vi "test_F9P-fgv.vi"() -> ()   [LabVIEW 2019]
uses:
  Ctrl/gnss_config.ctl
panel:
  out "error out":errorcluster
  out "read_buffer":string
  in  "GNSS cfg":T1={"Port"="COM10", "heading select"="", "PwrPak7_mode select"=[], "rate"=115200}
  out "UTM graph":cluster{"X":dbl, "Y":dbl}[](graph)=[{"X"=161777.95400057395, "Y"=515289.5740891766}, {"X"=161777.91880889426, "Y"=515289.640840397}, {"X"=161777.91926328043, "Y"=515289.74072502257}, {"X"=161777.89309671233, "Y"=515289.8407307517}, {"X"=161777.83123359273, "Y"=515289.89650478243}, {"X"=161777.8049155659, "Y"=515289.96321563463}, {"X"=161777.78731972742, "Y"=515289.99659124424}, {"X"=161777.7073558953, "Y"=515289.97475796775}, {"X"=161777.6717603178, "Y"=515289.95272285305}, {"X"=161777.59169550939, "Y"=515289.90869299456}, {"X"=161777.53835263004, "Y"=515289.8867386161}, {"X"=161777.5565543218, "Y"=515289.98654250597}, {"X"=161777.94820664724, "Y"=515290.2511253461}, {"X"=161778.5442558229, "Y"=515290.58136952063}, {"X"=161779.19379927934, "Y"=515290.9668630023}, {"X"=161779.82615070668, "Y"=515291.4745184741}, {"X"=161780.5468851608, "Y"=515291.90408230544}, {"X"=161781.3293312115, "Y"=515292.24457731773}, {"X"=161782.0763330891, "Y"=515292.5963321432}, {"X"=161782.7433711131, "Y"=515292.92625371326}, {"X"=161783.43763578677, "Y"=515293.3892337531}, {"X"=161784.1312441562, "Y"=515293.707936055}, {"X"=161784.81607978063, "Y"=515294.04887535865}, {"X"=161785.45700141956, "Y"=515294.4899011407}, {"X"=161786.09792298873, "Y"=515294.93092697154}, {"X"=161786.7387940146, "Y"=515295.3608545599}, {"X"=161787.44137668586, "Y"=515295.70171335887}, {"X"=161788.13513613178, "Y"=515296.0537108666}, {"X"=161788.81114823182, "Y"=515296.4057891417}, {"X"=161789.51388214662, "Y"=515296.7799429905}, {"X"=161790.16377791404, "Y"=515297.24312535825}, {"X"=161790.75927092956, "Y"=515297.4512891845}, {"X"=161791.45222257613, "Y"=515297.6257142923}, {"X"=161792.2164661421, "Y"=515297.8664063941}, {"X"=161792.9802554574, "Y"=515298.00721393456}, {"X"=161793.57564741094, "Y"=515298.1931813774}, {"X"=161794.04680835863, "Y"=515298.3797137626}, {"X"=161794.66105778705, "Y"=515298.8097630031}, {"X"=161795.2851396199, "Y"=515299.4506394842}, {"X"=161795.79295568907, "Y"=515299.8922712862}, {"X"=161796.44179114, "Y"=515300.1223900075}, {"X"=161797.13539845136, "Y"=515300.4410933779}, {"X"=161797.67023897104, "Y"=515300.97139058786}, {"X"=161798.35436699775, "Y"=515301.1569549014}, {"X"=161799.0217064507, "Y"=515301.5534675081}, {"X"=161799.63580401638, "Y"=515301.95022223337}, {"X"=161800.4886824086, "Y"=515302.168315055}, {"X"=161801.34135892912, "Y"=515302.3420147952}, {"X"=161802.02755544466, "Y"=515302.98260937684}, {"X"=161802.80137821336, "Y"=515303.37863818085}, {"X"=161803.5310850009, "Y"=515303.83036021655}, {"X"=161804.18138306442, "Y"=515304.3823299997}, {"X"=161804.83979789636, "Y"=515304.7677851127}, {"X"=161805.60444402587, "Y"=515305.0972647629}, {"X"=161806.39525694898, "Y"=515305.3267388399}, {"X"=161807.21314476756, "Y"=515305.6559766089}, {"X"=161807.87039905335, "Y"=515305.7861712441}, {"X"=161808.54550148163, "Y"=515305.9384818447}, {"X"=161809.22151191556, "Y"=515306.29056175554}, {"X"=161809.90669859963, "Y"=515306.70919113874}, {"X"=161810.5830115807, "Y"=515307.12786090834}, {"X"=161811.30308733214, "Y"=515307.41314957023}, {"X"=161812.0322888786, "Y"=515307.7538894202}, {"X"=161812.72589495758, "Y"=515308.0725940717}, {"X"=161813.28574078486, "Y"=515308.2476259363}, {"X"=161813.93437333827, "Y"=515308.43335283204}, {"X"=161814.49391648162, "Y"=515308.54179502284}, {"X"=161814.78750287872, "Y"=515308.7069385592}, {"X"=161814.86736555945, "Y"=515308.70657560363}, {"X"=161814.89428908148, "Y"=515308.7730443711}, {"X"=161814.89474303092, "Y"=515308.87292899843}, {"X"=161814.9569593225, "Y"=515308.89484328456}, {"X"=161814.98358021321, "Y"=515308.8947222998}, {"X"=161815.0456956249, "Y"=515308.89444000245}, {"X"=161815.0901646555, "Y"=515308.9164349459}, {"X"=161815.14370907008, "Y"=515308.9827827293}, {"X"=161815.2241770044, "Y"=515309.1155992807}, {"X"=161815.30444318076, "Y"=515309.2040226664}, {"X"=161815.39373430205, "Y"=515309.3257005998}, {"X"=161815.4736978485, "Y"=515309.34753423324}, {"X"=161815.52704050532, "Y"=515309.36948885216}, {"X"=161815.58033272164, "Y"=515309.38034517795}, {"X"=161815.64270031895, "Y"=515309.4355543454}, {"X"=161815.68711890728, "Y"=515309.44645099895}, {"X"=161815.7316888065, "Y"=515309.4906425299}, {"X"=161815.7674355156, "Y"=515309.54597268056}, {"X"=161815.8119549762, "Y"=515309.57906591985}, {"X"=161815.85632312373, "Y"=515309.57886428316}, {"X"=161815.89186808158, "Y"=515309.58980126516}, {"X"=161815.92741303705, "Y"=515309.6007382487}, {"X"=161815.95398349033, "Y"=515309.5895189744}, {"X"=161815.90916140308, "Y"=515309.48983598285}, {"X"=161815.93598404175, "Y"=515309.5341081699}, {"X"=161815.95378174057, "Y"=515309.54512580705}, {"X"=161815.97147856222, "Y"=515309.53394686105}, {"X"=161815.98040262918, "Y"=515309.54500482546}, {"X"=161816.0160988968, "Y"=515309.58923668414}, {"X"=161816.06076966808, "Y"=515309.65562480193}, {"X"=161816.18520223314, "Y"=515309.6994533913}, {"X"=161816.22982256542, "Y"=515309.754743216}, {"X"=161816.26521620865, "Y"=515309.73238532426}, {"X"=161816.30055941732, "Y"=515309.6989291415}, {"X"=161816.32738205325, "Y"=515309.74320132786}, {"X"=161816.18449611322, "Y"=515309.5440773027}, {"X"=161816.11305313953, "Y"=515309.4445152901}, {"X"=161816.13080039885, "Y"=515309.44443463604}, {"X"=161816.14885028123, "Y"=515309.51094373537}, {"X"=161816.1668497262, "Y"=515309.5663545408}, {"X"=161816.25639301635, "Y"=515309.7435239428}, {"X"=161816.51468657114, "Y"=515309.95322201477}, {"X"=161817.0042996991, "Y"=515310.29505111795}, {"X"=161817.65373897512, "Y"=515310.65835097386}, {"X"=161818.44465190032, "Y"=515310.9100227651}, {"X"=161819.26248826162, "Y"=515311.2281634111}, {"X"=161820.07099704226, "Y"=515311.44645983004}, {"X"=161820.90537020008, "Y"=515311.49816098064}, {"X"=161821.74896998494, "Y"=515311.6275099376}, {"X"=161822.53917668908, "Y"=515311.723806025}, {"X"=161823.3205601771, "Y"=515311.83124079654}, {"X"=161824.10229662905, "Y"=515312.01636368537}, {"X"=161824.87546197322, "Y"=515312.2681167172}, {"X"=161825.6757019711, "Y"=515312.6196334966}, {"X"=161826.44004401113, "Y"=515312.8825252806}, {"X"=161827.20433557767, "Y"=515313.13431884075}, {"X"=161828.02186885226, "Y"=515313.38587058336}, {"X"=161828.82180608835, "Y"=515313.6707979099}, {"X"=161829.66601055447, "Y"=515313.9333271637}, {"X"=161830.48324116512, "Y"=515314.11828939256}, {"X"=161831.35401598827, "Y"=515314.3695995875}, {"X"=161832.19837155048, "Y"=515314.665423971}, {"X"=161833.016559914, "Y"=515315.0612539941}, {"X"=161833.74565907218, "Y"=515315.37979913654}, {"X"=161834.43921326537, "Y"=515315.68740728305}, {"X"=161835.15933786728, "Y"=515315.9837962724}, {"X"=161835.89726006903, "Y"=515316.2912030018}, {"X"=161836.63518221842, "Y"=515316.598609796}, {"X"=161837.37320513173, "Y"=515316.9282132381}, {"X"=161838.10245518197, "Y"=515317.2800536338}, {"X"=161838.8584268477, "Y"=515317.65396976646}, {"X"=161839.62352409755, "Y"=515318.083337126}, {"X"=161840.30830503887, "Y"=515318.4131826406}, {"X"=161841.0286812179, "Y"=515318.76506358985}, {"X"=161841.77557738448, "Y"=515319.09462711634}, {"X"=161842.54042233957, "Y"=515319.46850327816}, {"X"=161843.24350470793, "Y"=515319.9203496465}, {"X"=161843.9554606182, "Y"=515320.3721557716}, {"X"=161844.631921982, "Y"=515320.82412314625}, {"X"=161845.31725688517, "Y"=515321.2760502795}, {"X"=161846.07312706957, "Y"=515321.6277704748}, {"X"=161846.81967000206, "Y"=515321.8796464045}, {"X"=161847.59273294985, "Y"=515322.1092049326}, {"X"=161848.31280612783, "Y"=515322.3944967517}, {"X"=161849.10391857562, "Y"=515322.6905645844}, {"X"=161849.85025974846, "Y"=515322.8980476132}, {"X"=161850.52480569232, "Y"=515322.92828036164}, {"X"=161851.28864208458, "Y"=515323.0801914752}, {"X"=161852.08802329528, "Y"=515323.24303979415}, {"X"=161852.87011074505, "Y"=515323.5058533946}, {"X"=161853.64337491884, "Y"=515323.7798056455}, {"X"=161854.3632461972, "Y"=515324.02070481237}, {"X"=161855.10988943258, "Y"=515324.2947780592}, {"X"=161855.89222861396, "Y"=515324.61308340123}, {"X"=161856.67471888705, "Y"=515324.9646836894}, {"X"=161857.47475478542, "Y"=515325.27181031683}, {"X"=161858.2394473211, "Y"=515325.61239302583}, {"X"=161858.96017477982, "Y"=515326.0419635504}, {"X"=161859.69834711196, "Y"=515326.40486382256}, {"X"=161860.5074578888, "Y"=515326.7563436241}, {"X"=161861.28954474037, "Y"=515327.0191580045}, {"X"=161862.02746499534, "Y"=515327.32656702003}, {"X"=161862.76538520248, "Y"=515327.63397609856}, {"X"=161863.53002692718, "Y"=515327.9634609943}, {"X"=161864.29471896973, "Y"=515328.30404425325}, {"X"=161865.06818381284, "Y"=515328.6223907203}, {"X"=161865.84164859212, "Y"=515328.94073725946}, {"X"=161866.57049341834, "Y"=515329.20379377867}, {"X"=161867.33488300277, "Y"=515329.47778755915}, {"X"=161868.09937327213, "Y"=515329.7739779929}, {"X"=161868.82877200074, "Y"=515330.1591159194}, {"X"=161869.56709463586, "Y"=515330.5553119311}, {"X"=161870.3317861905, "Y"=515330.8958957367}, {"X"=161871.06133581288, "Y"=515331.31432873226}, {"X"=161871.80873330153, "Y"=515331.7548778398}, {"X"=161872.52078738002, "Y"=515332.22888295737}, {"X"=161873.2063716484, "Y"=515332.73630381504}, {"X"=161873.8827800619, "Y"=515333.1771752419}, {"X"=161874.57688525325, "Y"=515333.60686789843}, {"X"=161875.27094001378, "Y"=515334.02546231856}, {"X"=161876.06215110896, "Y"=515334.3437292654}, {"X"=161876.7820711783, "Y"=515334.59572863765}, {"X"=161877.53773739794, "Y"=515334.90305848164}, {"X"=161878.1777949538, "Y"=515335.15542033466}, {"X"=161878.83554931934, "Y"=515335.39660342183}, {"X"=161879.61758442305, "Y"=515335.6483212079}, {"X"=161880.42618993216, "Y"=515335.8888199965}, {"X"=161881.31536272637, "Y"=515336.2843326286}, {"X"=161882.11595047737, "Y"=515336.713542806}, {"X"=161882.925109656, "Y"=515337.0761230474}, {"X"=161883.8140808093, "Y"=515337.42724277306}, {"X"=161884.68545573042, "Y"=515337.81173797994}, {"X"=161885.48589212738, "Y"=515338.2076535997}, {"X"=161886.30382391758, "Y"=515338.54799732764}, {"X"=161887.15694797394, "Y"=515338.8215903732}, {"X"=161888.00104734325, "Y"=515339.0619288787}, {"X"=161888.8096522778, "Y"=515339.3024284715}, {"X"=161889.6010133728, "Y"=515339.6539915637}, {"X"=161890.38329944562, "Y"=515339.96120180906}, {"X"=161891.20990310656, "Y"=515340.2571125954}, {"X"=161892.07245413205, "Y"=515340.65274710406}, {"X"=161892.88146147915, "Y"=515340.9820334242}, {"X"=161893.70801461404, "Y"=515341.266846164}, {"X"=161894.51687083603, "Y"=515341.562837765}, {"X"=161895.34337352356, "Y"=515341.8365523713}, {"X"=161896.16115355797, "Y"=515342.1436021796}, {"X"=161896.98760579992, "Y"=515342.40621865366}, {"X"=161897.78743720995, "Y"=515342.668955934}, {"X"=161898.53417799206, "Y"=515342.9652296072}, {"X"=161899.3162621102, "Y"=515343.2280475129}, {"X"=161900.21380354543, "Y"=515343.5125389749}, {"X"=161901.05800270947, "Y"=515343.77507537254}, {"X"=161901.87623526133, "Y"=515344.1820103629}, {"X"=161902.65867142286, "Y"=515344.52251662395}, {"X"=161903.405361544, "Y"=515344.8076924376}, {"X"=161904.1878982269, "Y"=515345.17039542255}, {"X"=161905.05009587965, "Y"=515345.48834321246}, {"X"=161905.8766481465, "Y"=515345.7731571441}, {"X"=161906.73864439924, "Y"=515346.04671193776}, {"X"=161907.60971545277, "Y"=515346.3646197568}, {"X"=161908.4986342502, "Y"=515346.70464379125}, {"X"=161909.352108935, "Y"=515347.05592712766}, {"X"=161910.17024013115, "Y"=515347.4406663381}, {"X"=161910.98811968672, "Y"=515347.7699141675}, {"X"=161911.8503671221, "Y"=515348.0989609433}, {"X"=161912.64142454168, "Y"=515348.3839364425}, {"X"=161913.3880636627, "Y"=515348.6580148472}, {"X"=161914.12643284362, "Y"=515349.06531304884}, {"X"=161914.9178925542, "Y"=515349.43907509785}, {"X"=161915.74479622993, "Y"=515349.80157804146}, {"X"=161916.60714387614, "Y"=515350.15282188874}, {"X"=161917.46954175117, "Y"=515350.51516411605}, {"X"=161918.32316657176, "Y"=515350.89974323724}, {"X"=161919.1765901063, "Y"=515351.2399292743}, {"X"=161920.00319161528, "Y"=515351.53584288084}, {"X"=161920.8120961968, "Y"=515351.84293529525}, {"X"=161921.55036413745, "Y"=515352.22803756245}, {"X"=161922.36829306814, "Y"=515352.56838478544}, {"X"=161923.10630938952, "Y"=515352.8979957256}, {"X"=161923.8533501241, "Y"=515353.26086139417}, {"X"=161924.66245557135, "Y"=515353.61234734603}, {"X"=161925.48013277317, "Y"=515353.89720341103}, {"X"=161926.25283849932, "Y"=515354.0490811027}, {"X"=161926.99937607578, "Y"=515354.3009641277}, {"X"=161927.7989036433, "Y"=515354.4971144997}, {"X"=161928.6692689521, "Y"=515354.6596484004}, {"X"=161929.57437423227, "Y"=515354.65554717765}, {"X"=161930.4700527705, "Y"=515354.5294050439}, {"X"=161931.31133327156, "Y"=515354.148243518}, {"X"=161932.00090811338, "Y"=515353.5790945927}, {"X"=161932.69925606335, "Y"=515352.9877089369}, {"X"=161933.32646459132, "Y"=515352.36335009336}, {"X"=161933.80226917754, "Y"=515351.6175935328}, {"X"=161934.15379337373, "Y"=515350.8613015468}, {"X"=161934.48792243574, "Y"=515350.18277802714}, {"X"=161934.7774322105, "Y"=515349.4489640703}, {"X"=161935.07556422258, "Y"=515348.6596184621}, {"X"=161935.4357108523, "Y"=515347.84779487306}, {"X"=161935.78728563793, "Y"=515347.10260125354}, {"X"=161936.13875992826, "Y"=515346.3352110685}, {"X"=161936.41939639655, "Y"=515345.6014373766}, {"X"=161936.79834631603, "Y"=515345.0225975819}, {"X"=161937.20311261978, "Y"=515344.2660645376}, {"X"=161937.66132166225, "Y"=515343.5536834864}, {"X"=161938.00362102268, "Y"=515342.71974383073}, {"X"=161938.31904828746, "Y"=515341.83043332514}, {"X"=161938.69654051441, "Y"=515340.9297431562}, {"X"=161938.78120414057, "Y"=515340.0303795257}, {"X"=161939.13237735824, "Y"=515339.1963997258}, {"X"=161939.5731412986, "Y"=515338.5506889347}, {"X"=161939.87112334048, "Y"=515337.7280486421}, {"X"=161940.1958770621, "Y"=515336.9385826464}, {"X"=161940.65418731276, "Y"=515336.2483983565}, {"X"=161941.0591052153, "Y"=515335.5251603874}, {"X"=161941.49014127353, "Y"=515334.69081893854}, {"X"=161941.94815012685, "Y"=515333.9340449724}, {"X"=161942.3971849206, "Y"=515333.15511464124}, {"X"=161942.7756331237, "Y"=515332.4652922189}, {"X"=161943.27841240127, "Y"=515331.79710369575}, {"X"=161943.71862409374, "Y"=515331.0293119262}, {"X"=161944.10604664683, "Y"=515330.36164595786}, {"X"=161944.46649656442, "Y"=515329.6164125417}, {"X"=161944.91533075334, "Y"=515328.7930891884}, {"X"=161945.24033664548, "Y"=515328.05911486375}, {"X"=161945.50302625427, "Y"=515327.2810287196}, {"X"=161945.81920890935, "Y"=515326.5581929054}, {"X"=161946.13569321425, "Y"=515325.901946852}, {"X"=161946.42500381247, "Y"=515325.12374017213}, {"X"=161946.79387539616, "Y"=515324.27858204907}, {"X"=161947.16269679094, "Y"=515323.422325654}, {"X"=161947.59413620055, "Y"=515322.67677087436}, {"X"=161948.03394667563, "Y"=515321.82019301516}, {"X"=161948.45601000654, "Y"=515320.96369555395}, {"X"=161948.71870014715, "Y"=515320.18560952466}, {"X"=161949.11429356097, "Y"=515319.3625275367}, {"X"=161949.4475204146, "Y"=515318.4842354148}, {"X"=161950.06470318564, "Y"=515317.6046573629}, {"X"=161950.54041074455, "Y"=515316.83670523297}, {"X"=161950.98939700832, "Y"=515316.04667710536}, {"X"=161951.40324067828, "Y"=515315.334497779}, {"X"=161951.7375736189, "Y"=515314.70036817004}, {"X"=161951.98296933615, "Y"=515314.0222472447}, {"X"=161952.30797643325, "Y"=515313.28827321855}, {"X"=161952.7038218216, "Y"=515312.520682873}, {"X"=161952.93177197044, "Y"=515311.9092320918}, {"X"=161953.03428522788, "Y"=515311.0319848771}, {"X"=161953.2798319342, "Y"=515310.38715886796}, {"X"=161953.6583825907, "Y"=515309.71953355806}, {"X"=161953.90362785343, "Y"=515309.0081178228}, {"X"=161954.28227913257, "Y"=515308.36268912524}, {"X"=161954.63471161335, "Y"=515307.80616731907}, {"X"=161954.7294570668, "Y"=515307.17312272196}, {"X"=161954.96552733905, "Y"=515306.3951574542}, {"X"=161955.21016977262, "Y"=515305.55056226446}, {"X"=161955.60576453415, "Y"=515304.7274806116}, {"X"=161955.59412698867, "Y"=515304.11711476854}, {"X"=161955.86584273542, "Y"=515303.37228368537}, {"X"=161956.1372570139, "Y"=515302.5608628645}, {"X"=161956.22212396463, "Y"=515301.7058926454}, {"X"=161955.96066780292, "Y"=515300.7969979573}, {"X"=161955.69084047474, "Y"=515299.9991263682}, {"X"=161955.191052268, "Y"=515299.36877383845}, {"X"=161954.68304364916, "Y"=515298.88273930375}, {"X"=161954.0248364, "Y"=515298.5416656653}, {"X"=161953.33103402163, "Y"=515298.1785562245}, {"X"=161952.65528040676, "Y"=515297.88195622247}, {"X"=161951.94423321, "Y"=515297.6299101742}, {"X"=161951.28537238724, "Y"=515297.14455896453}, {"X"=161950.61834147936, "Y"=515296.81462406786}, {"X"=161949.99593002838, "Y"=515296.539979752}, {"X"=161949.3458923907, "Y"=515296.04349021724}, {"X"=161948.69615624959, "Y"=515295.6135904783}, {"X"=161948.04672161583, "Y"=515295.2502805372}, {"X"=161947.38821222726, "Y"=515294.84261766996}, {"X"=161946.76539840753, "Y"=515294.4791872635}, {"X"=161946.08087114274, "Y"=515294.204824559}, {"X"=161945.36927050393, "Y"=515293.8306978602}, {"X"=161944.6758694966, "Y"=515293.55637546064}, {"X"=161943.90240455308, "Y"=515293.23802168}, {"X"=161943.18142739666, "Y"=515292.752952447}, {"X"=161942.48707109463, "Y"=515292.26776269486}, {"X"=161941.80123646528, "Y"=515291.704844767}, {"X"=161941.0711843177, "Y"=515291.175422743}, {"X"=161940.27064561704, "Y"=515290.75730525906}, {"X"=161939.48815577972, "Y"=515290.4056972044}, {"X"=161938.72351372213, "Y"=515290.07620541175}, {"X"=161938.00374261462, "Y"=515289.85749560664}, {"X"=161937.27524864773, "Y"=515289.67212093744}, {"X"=161936.58169619142, "Y"=515289.36450432875}, {"X"=161935.81750643376, "Y"=515289.13489741914}, {"X"=161935.06219028393, "Y"=515288.90525037656}, {"X"=161934.27148005128, "Y"=515288.69796079333}, {"X"=161933.41068564297, "Y"=515288.69076214795}, {"X"=161932.6569784392, "Y"=515288.8162606383}, {"X"=161931.8672235296, "Y"=515288.8198388122}, {"X"=161931.07711662684, "Y"=515288.74572902126}, {"X"=161930.3219008794, "Y"=515288.5382789876}, {"X"=161929.47739542314, "Y"=515288.20914988924}, {"X"=161928.65951085434, "Y"=515287.87990024895}, {"X"=161927.9568831186, "Y"=515287.5279313939}, {"X"=161927.2716506, "Y"=515287.09819413896}, {"X"=161926.5866191725, "Y"=515286.71285010525}, {"X"=161925.86609307144, "Y"=515286.3276669711}, {"X"=161925.14561719442, "Y"=515285.9535821874}, {"X"=161924.3721005021, "Y"=515285.62413190625}, {"X"=161923.5722645573, "Y"=515285.3613920831}, {"X"=161922.73693393928, "Y"=515285.09881319216}, {"X"=161921.98141587077, "Y"=515284.8247741575}, {"X"=161921.19922648455, "Y"=515284.5397575458}, {"X"=161920.4792029357, "Y"=515284.2655577826}, {"X"=161919.7587266356, "Y"=515283.89147346036}, {"X"=161918.98515923883, "Y"=515283.55092538125}, {"X"=161918.2112899671, "Y"=515283.14378762734}, {"X"=161917.42869787168, "Y"=515282.7699850365}, {"X"=161916.6461560055, "Y"=515282.40728080965}, {"X"=161915.9078314518, "Y"=515282.0110806749}, {"X"=161915.18730444807, "Y"=515281.62589845166}, {"X"=161914.4407097777, "Y"=515281.3629181606}, {"X"=161913.70308933442, "Y"=515281.1220942942}, {"X"=161913.00076224905, "Y"=515280.8367164303}, {"X"=161912.32495547645, "Y"=515280.5290213668}, {"X"=161911.5425641136, "Y"=515280.19961248635}, {"X"=161910.75155058503, "Y"=515279.9257353611}, {"X"=161909.96931004123, "Y"=515279.6296214994}, {"X"=161909.159945319, "Y"=515279.22264548496}, {"X"=161908.25302055696, "Y"=515278.82721036416}, {"X"=161907.33717173082, "Y"=515278.42071727884}, {"X"=161906.4481953906, "Y"=515278.0695950546}, {"X"=161905.57696629775, "Y"=515277.71839245874}, {"X"=161904.71521463455, "Y"=515277.5003292154}, {"X"=161903.87983230813, "Y"=515277.2266538999}, {"X"=161903.062096607, "Y"=515276.9307016142}, {"X"=161902.2795032462, "Y"=515276.5569004291}, {"X"=161901.47941410658, "Y"=515276.2386712453}, {"X"=161900.67922425573, "Y"=515275.8982455542}, {"X"=161899.88780734973, "Y"=515275.53558311897}, {"X"=161899.1048110966, "Y"=515275.0729958998}, {"X"=161898.26917670213, "Y"=515274.74382968387}, {"X"=161897.477910569, "Y"=515274.41446234775}, {"X"=161896.6331507237, "Y"=515274.02984508174}, {"X"=161895.80618846533, "Y"=515273.65624570387}, {"X"=161894.9967721373, "Y"=515273.2381727572}, {"X"=161894.1519113932, "Y"=515272.8313591558}, {"X"=161893.26278289093, "Y"=515272.4469434479}, {"X"=161892.32958797965, "Y"=515272.12931881077}, {"X"=161891.50358174255, "Y"=515271.96658738586}, {"X"=161890.70369309804, "Y"=515271.6927523866}, {"X"=161889.87662966445, "Y"=515271.29695700866}, {"X"=161889.03166778968, "Y"=515270.86794733745}, {"X"=161888.19593188778, "Y"=515270.51658553944}, {"X"=161887.3959423095, "Y"=515270.2205542715}, {"X"=161886.58702865976, "Y"=515269.91346504155}, {"X"=161885.7782156393, "Y"=515269.62857247214}, {"X"=161884.9958725429, "Y"=515269.3102643434}, {"X"=161884.20465571477, "Y"=515268.9919965427}, {"X"=161883.5019741573, "Y"=515268.62893309694}, {"X"=161882.73732787618, "Y"=515268.2994463761}, {"X"=161881.99925220365, "Y"=515267.95874066214}, {"X"=161881.21695915365, "Y"=515267.6515311742}, {"X"=161880.3907004909, "Y"=515267.4333093851}, {"X"=161879.56429072845, "Y"=515267.1817927991}, {"X"=161878.87078461153, "Y"=515266.88527922577}, {"X"=161878.21257172697, "Y"=515266.5442115003}, {"X"=161877.50983934605, "Y"=515266.1700502625}, {"X"=161876.736218213, "Y"=515265.8184077638}, {"X"=161875.98896625204, "Y"=515265.41115309286}, {"X"=161875.2595622916, "Y"=515265.0260145416}, {"X"=161874.47701692148, "Y"=515264.66331422405}, {"X"=161873.66790080853, "Y"=515264.3118330678}, {"X"=161872.85903643933, "Y"=515264.01584344613}, {"X"=161872.0765915923, "Y"=515263.6753399338}, {"X"=161871.28517227838, "Y"=515263.3126801803}, {"X"=161870.59111153655, "Y"=515262.89408608596}, {"X"=161869.8352875275, "Y"=515262.55346197344}, {"X"=161869.01759953576, "Y"=515262.2686112796}, {"X"=161868.29742122997, "Y"=515261.96112109604}, {"X"=161867.57739397406, "Y"=515261.6869258457}, {"X"=161866.80447717488, "Y"=515261.49066033296}, {"X"=161866.0137122376, "Y"=515261.27227885707}, {"X"=161865.27613897348, "Y"=515261.04255751584}, {"X"=161864.51184387924, "Y"=515260.7907604823}, {"X"=161863.77416977895, "Y"=515260.5388426918}, {"X"=161863.00972346903, "Y"=515260.2537509228}, {"X"=161862.20948012735, "Y"=515259.90223058756}, {"X"=161861.46247880755, "Y"=515259.5504686582}, {"X"=161860.74219923108, "Y"=515259.22078253725}, {"X"=161860.03124668341, "Y"=515258.990940815}, {"X"=161859.31242800006, "Y"=515258.98310525273}, {"X"=161858.717740113, "Y"=515258.9525092296}, {"X"=161858.16716873465, "Y"=515258.8662203797}, {"X"=161857.52871700065, "Y"=515258.969005343}, {"X"=161856.8642992053, "Y"=515259.21618898667}, {"X"=161856.27964382304, "Y"=515259.4408135441}, {"X"=161855.83636278144, "Y"=515259.5316140942}, {"X"=161855.63221770368, "Y"=515259.5214423518}, {"X"=161855.596823744, "Y"=515259.5438000729}, {"X"=161855.57897560915, "Y"=515259.5216840613}, {"X"=161855.54343049665, "Y"=515259.51074691024}, {"X"=161855.5344560482, "Y"=515259.48859061324}, {"X"=161855.4899868667, "Y"=515259.4665954573}, {"X"=161855.45429059828, "Y"=515259.4223634318}, {"X"=161855.41864471624, "Y"=515259.3892297002}, {"X"=161855.3918221316, "Y"=515259.3449573912}, {"X"=161855.3561258644, "Y"=515259.30072536797}, {"X"=161855.33817695922, "Y"=515259.2564127754}, {"X"=161855.31115283526, "Y"=515259.1677473023}, {"X"=161855.26648211508, "Y"=515259.10135898314}, {"X"=161855.21318963537, "Y"=515259.0905024035}, {"X"=161855.19534149853, "Y"=515259.06838639313}, {"X"=161855.1775941335, "Y"=515259.0684669638}, {"X"=161855.1597459988, "Y"=515259.0463509517}, {"X"=161855.141897864, "Y"=515259.02423494007}, {"X"=161855.1329737943, "Y"=515259.01317693456}, {"X"=161855.13287302462, "Y"=515258.9909803531}, {"X"=161855.13277225487, "Y"=515258.9687837711}, {"X"=161855.13277225487, "Y"=515258.9687837711}, {"X"=161855.14159555495, "Y"=515258.95764519426}, {"X"=161855.1415451701, "Y"=515258.9465469033}, {"X"=161855.13262110035, "Y"=515258.93548889866}, {"X"=161855.12364664793, "Y"=515258.9133326021}, {"X"=161855.12359626306, "Y"=515258.90223430976}, {"X"=161855.12344510847, "Y"=515258.8689394378}, {"X"=161855.13216763665, "Y"=515258.8356042799}, {"X"=161855.140940552, "Y"=515258.8133674116}, {"X"=161855.14976384997, "Y"=515258.8022288338}, {"X"=161855.1496630803, "Y"=515258.7800322537}, {"X"=161855.16730967636, "Y"=515258.7577550996}, {"X"=161855.1760825896, "Y"=515258.7355182323}, {"X"=161855.18485550067, "Y"=515258.7132813659}, {"X"=161855.19357803153, "Y"=515258.67994620814}, {"X"=161855.193477262, "Y"=515258.6577496248}, {"X"=161855.19337649245, "Y"=515258.63555304374}, {"X"=161855.1308576305, "Y"=515258.5470487136}, {"X"=161855.12158086852, "Y"=515258.4583026712}, {"X"=161855.16584851703, "Y"=515258.43590466277}, {"X"=161855.15727714272, "Y"=515258.5025346935}, {"X"=161855.13075686077, "Y"=515258.5248521298}, {"X"=161855.139680931, "Y"=515258.5359101363}, {"X"=161855.14845384442, "Y"=515258.5136732685}, {"X"=161855.13952977647, "Y"=515258.50261526427}, {"X"=161855.1039342742, "Y"=515258.4805798231}, {"X"=161855.0951109737, "Y"=515258.4917184}, {"X"=161855.07741399008, "Y"=515258.50289726234}, {"X"=161855.06874184893, "Y"=515258.54733071174}, {"X"=161855.08583421126, "Y"=515258.4029723567}, {"X"=161855.04096194322, "Y"=515258.2921908753}, {"X"=161855.04983562883, "Y"=515258.29215058975}, {"X"=161855.04101232818, "Y"=515258.30328916764}, {"X"=161855.01444166317, "Y"=515258.3145083138}, {"X"=161855.01449204815, "Y"=515258.3256066038}, {"X"=161855.02346650147, "Y"=515258.3477629017}, {"X"=161855.02341611648, "Y"=515258.33666460926}, {"X"=161855.01464320318, "Y"=515258.3589014782}, {"X"=161855.01474397315, "Y"=515258.3810980592}, {"X"=161855.0148447432, "Y"=515258.40329464065}, {"X"=161855.02391996636, "Y"=515258.4476475195}, {"X"=161854.99739968686, "Y"=515258.4699649585}, {"X"=161854.97945078035, "Y"=515258.4256523657}, {"X"=161854.94435912828, "Y"=515258.514599835}, {"X"=161854.90009148075, "Y"=515258.5369978455}, {"X"=161854.78463282995, "Y"=515258.5153249774}, {"X"=161854.69564406716, "Y"=515258.46023638215}, {"X"=161854.66877109034, "Y"=515258.4048657835}, {"X"=161854.6599477926, "Y"=515258.41600436135}, {"X"=161854.57948001442, "Y"=515258.28318744176}, {"X"=161854.13352846014, "Y"=515257.7857786603}, {"X"=161853.5367242136, "Y"=515257.28905478073}, {"X"=161852.82536819577, "Y"=515256.97042733885}, {"X"=161852.086887182, "Y"=515256.5409379131}, {"X"=161851.34003630254, "Y"=515256.2224717519}, {"X"=161850.50454928636, "Y"=515255.92660514}, {"X"=161849.5445786382, "Y"=515255.5758112337}, {"X"=161848.61067464348, "Y"=515255.1028153595}, {"X"=161847.66835040954, "Y"=515254.7297445006}, {"X"=161846.74352148225, "Y"=515254.3011017022}, {"X"=161845.85373364337, "Y"=515253.77241320733}, {"X"=161845.04380889304, "Y"=515253.2433621412}, {"X"=161844.41009785637, "Y"=515252.43604794407}, {"X"=161843.6972794797, "Y"=515251.7955708352}, {"X"=161842.904295368, "Y"=515251.08886672417}, {"X"=161842.20897213925, "Y"=515250.3928176908}, {"X"=161841.57566383813, "Y"=515249.6742900328}, {"X"=161841.06764560664, "Y"=515249.18826232955}, {"X"=161840.44351323618, "Y"=515248.53628420434}, {"X"=161839.7481391884, "Y"=515247.82913708314}, {"X"=161839.11488089088, "Y"=515247.12170790124}, {"X"=161838.3936416237, "Y"=515246.58115616144}, {"X"=161837.67245267576, "Y"=515246.05170277384}, {"X"=161836.98645597082, "Y"=515245.4554984823}, {"X"=161836.33590355213, "Y"=515244.8480347374}, {"X"=161835.59706774977, "Y"=515244.3408587182}, {"X"=161834.69895897733, "Y"=515243.934292904}, {"X"=161833.93345148241, "Y"=515243.41613966104}, {"X"=161833.15937267244, "Y"=515242.96461653925}, {"X"=161832.2437178918, "Y"=515242.60252476716}, {"X"=161831.30250066926, "Y"=515242.4736181307}, {"X"=161830.52847204602, "Y"=515242.0331935415}, {"X"=161829.80950059928, "Y"=515241.99206562154}, {"X"=161829.00940536047, "Y"=515241.67384330614}, {"X"=161828.2088562769, "Y"=515241.25573645125}, {"X"=161827.3732156748, "Y"=515240.92657725624}, {"X"=161826.63503446712, "Y"=515240.56367980246}, {"X"=161825.8443169042, "Y"=515240.3564003808}, {"X"=161824.97318130618, "Y"=515240.0274026874}, {"X"=161824.16370773275, "Y"=515239.5982382425}, {"X"=161823.31006726323, "Y"=515239.21366863215}, {"X"=161822.66747937835, "Y"=515238.4063963865}, {"X"=161821.90262619706, "Y"=515238.0325220135}, {"X"=161821.01389407594, "Y"=515237.7369002411}, {"X"=161820.1167924954, "Y"=515237.5523017953}, {"X"=161819.2818572464, "Y"=515237.3785194732}, {"X"=161818.43719089558, "Y"=515237.01610661217}, {"X"=161817.67243826826, "Y"=515236.66442920547}, {"X"=161816.90818992147, "Y"=515236.4237347723}, {"X"=161816.10784146975, "Y"=515236.0500222286}, {"X"=161815.32554298593, "Y"=515235.7428188506}, {"X"=161814.4638350129, "Y"=515235.5358631125}, {"X"=161813.69852724997, "Y"=515235.0621048665}, {"X"=161812.88900217068, "Y"=515234.621843212}, {"X"=161812.0888551327, "Y"=515234.29252421064}, {"X"=161811.2793803383, "Y"=515233.8633610007}, {"X"=161810.2504335617, "Y"=515233.9568258459}, {"X"=161809.3925086419, "Y"=515234.58224243444}, {"X"=161808.8284755823, "Y"=515235.4393921917}, {"X"=161808.40637150634, "Y"=515236.2847983398}, {"X"=161807.8515150515, "Y"=515237.208497576}, {"X"=161807.3230780444, "Y"=515238.08768267825}, {"X"=161806.78571699423, "Y"=515238.95580986154}, {"X"=161806.14131667535, "Y"=515239.7023399258}, {"X"=161805.71038983687, "Y"=515240.5588848489}, {"X"=161805.24391782834, "Y"=515241.40449285484}, {"X"=161804.83104127852, "Y"=515242.32754689525}, {"X"=161804.4093920267, "Y"=515243.27283787885}, {"X"=161804.10315140334, "Y"=515244.22870276636}, {"X"=161803.68125006903, "Y"=515245.11850233603}, {"X"=161803.29504542265, "Y"=515246.05253373215}, {"X"=161802.81964982036, "Y"=515246.88708393427}, {"X"=161802.3532793717, "Y"=515247.75488869747}, {"X"=161801.90465641086, "Y"=515248.6226128033}, {"X"=161801.45653809985, "Y"=515249.60131984786}, {"X"=161801.10577822817, "Y"=515250.52409169497}, {"X"=161800.57709049882, "Y"=515251.3477857985}, {"X"=161800.0303527461, "Y"=515252.104970874}, {"X"=161799.59927580992, "Y"=515252.92822126206}, {"X"=161799.13250236766, "Y"=515253.70723988744}, {"X"=161798.7812383369, "Y"=515254.5190289297}, {"X"=161798.33246473613, "Y"=515255.35345837043}, {"X"=161797.84809556048, "Y"=515256.165852635}, {"X"=161797.3906502994, "Y"=515257.0447156392}, {"X"=161796.97727078875, "Y"=515257.8567871894}, {"X"=161796.4749526731, "Y"=515258.6248690677}, {"X"=161796.07957301257, "Y"=515259.4923514257}, {"X"=161795.737334596, "Y"=515260.33739513234}, {"X"=161795.52794914786, "Y"=515261.12634217145}, {"X"=161795.43382065525, "Y"=515261.8925681029}, {"X"=161795.24243495756, "Y"=515262.7369259113}, {"X"=161795.01560504647, "Y"=515263.59254341305}, {"X"=161794.9664505922, "Y"=515264.4917471048}, {"X"=161794.7931656082, "Y"=515265.41371226904}, {"X"=161794.6728703964, "Y"=515266.2799438849}, {"X"=161794.38392492334, "Y"=515267.13584385463}, {"X"=161794.2194128052, "Y"=515268.03557210235}, {"X"=161793.93031604623, "Y"=515268.85817721806}, {"X"=161793.59730517826, "Y"=515269.7808687173}, {"X"=161793.15760846826, "Y"=515270.65965127945}, {"X"=161792.77100246848, "Y"=515271.5048968799}, {"X"=161792.44681504043, "Y"=515272.4164497904}, {"X"=161792.0958552752, "Y"=515273.29482889466}, {"X"=161791.80670844193, "Y"=515274.106335799}, {"X"=161791.48201653123, "Y"=515274.90690583625}, {"X"=161791.24686885078, "Y"=515275.88464502105}, {"X"=161790.99392343074, "Y"=515276.8513666277}, {"X"=161790.62471197709, "Y"=515277.6188435934}, {"X"=161790.09567372166, "Y"=515278.3648503689}, {"X"=161789.89607142366, "Y"=515279.353526472}, {"X"=161789.8119277122, "Y"=515280.3638745571}, {"X"=161789.80704129825, "Y"=515281.2406799489}, {"X"=161789.8646238027, "Y"=515282.1948909054}, {"X"=161789.8063440289, "Y"=515283.0386435541}, {"X"=161789.79218019245, "Y"=515283.8267029737}, {"X"=161789.8671062258, "Y"=515284.69204688893}, {"X"=161789.9499974153, "Y"=515285.3575812015}, {"X"=161789.91773296622, "Y"=515286.0680332886}, {"X"=161789.7884135151, "Y"=515286.90101048927}, {"X"=161789.6580341875, "Y"=515287.50092356396}, {"X"=161789.6332302126, "Y"=515287.9005831325}, {"X"=161789.46740677013, "Y"=515288.5117559215}, {"X"=161788.85946544315, "Y"=515289.468993534}, {"X"=161788.00154782206, "Y"=515290.0944124185}, {"X"=161787.15048497802, "Y"=515290.2758593617}, {"X"=161786.2537920066, "Y"=515290.1800508866}, {"X"=161785.38301328194, "Y"=515289.92874534486}, {"X"=161784.62723861728, "Y"=515289.5992271674}, {"X"=161783.85356515174, "Y"=515289.23649490444}, {"X"=161783.03587672234, "Y"=515288.95165256626}, {"X"=161782.18223929385, "Y"=515288.567087126}, {"X"=161781.3199805482, "Y"=515288.23805359856}, {"X"=161780.50158515852, "Y"=515287.7978354193}, {"X"=161779.65732599568, "Y"=515287.52421279124}, {"X"=161778.86600578777, "Y"=515287.1837583005}, {"X"=161778.0211911494, "Y"=515286.7880546263}, {"X"=161777.2654663978, "Y"=515286.4696353992}, {"X"=161776.68807299162, "Y"=515286.3390798307}, {"X"=161776.59051327794, "Y"=515286.3506221759}, {"X"=161776.5997908469, "Y"=515286.43936814205}, {"X"=161776.58259891806, "Y"=515286.56153008796}, {"X"=161776.5828513634, "Y"=515286.6170215483}, {"X"=161776.59162403713, "Y"=515286.5947845961}, {"X"=161776.5652050334, "Y"=515286.63929886813}, {"X"=161776.57443211103, "Y"=515286.7169465434}, {"X"=161776.59253284012, "Y"=515286.79455384833}, {"X"=161776.60226481006, "Y"=515286.98318444006}, {"X"=161776.60302214575, "Y"=515287.1496588164}, {"X"=161776.60362801436, "Y"=515287.2828383192}, {"X"=161776.60403192675, "Y"=515287.3716246535}, {"X"=161776.58699146722, "Y"=515287.52708147664}, {"X"=161776.56112784226, "Y"=515287.6936769579}, {"X"=161776.54439031685, "Y"=515287.9157235328}, {"X"=161776.5361225362, "Y"=515288.0489434029}, {"X"=161776.53687987349, "Y"=515288.2154177806}, {"X"=161776.52004137615, "Y"=515288.41526777105}, {"X"=161776.51202603796, "Y"=515288.6039791006}, {"X"=161776.49493509153, "Y"=515288.7483376326}, {"X"=161776.47809659422, "Y"=515288.9481876227}, {"X"=161776.43468763283, "Y"=515289.1592570118}, {"X"=161776.4001523249, "Y"=515289.37028603186}, {"X"=161776.4008591759, "Y"=515289.52566211735}]
  in  "정지":bool
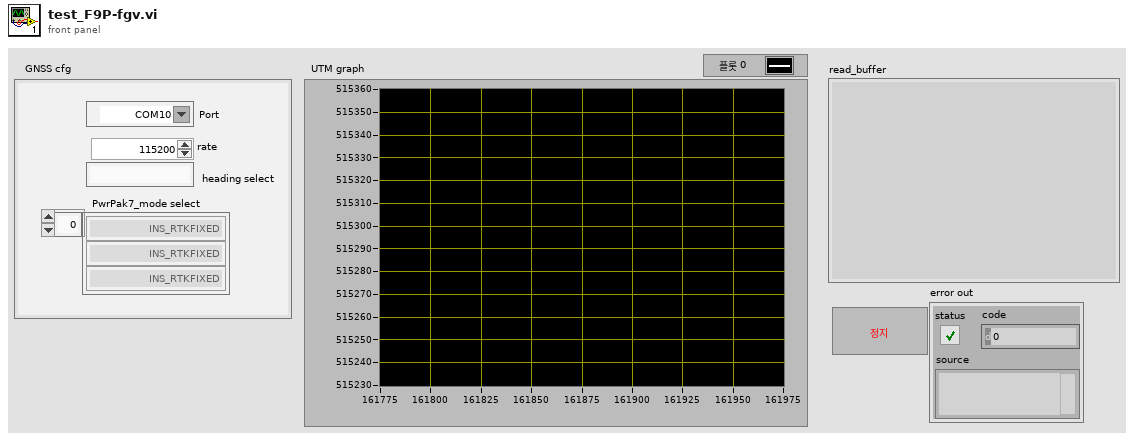
[diagram p1: front panel]
types:
  T1 = typedef "gnss_config.ctl" = cluster{"Port":refnum<visa-resource-name>, "heading select":string, "PwrPak7_mode select":string[], "rate":u32}
  T2 = enum16{"GxDTM", "GxGBS", "GxGGA", "GxGLL", "GxGNS", "GxGRS", "GxGSA", "GxGST", "GxGSV", "GxRLM", "GxRMC", "GxTHS", "GxTXT", "GxVLW", "GxVTG", "GxZDA"}
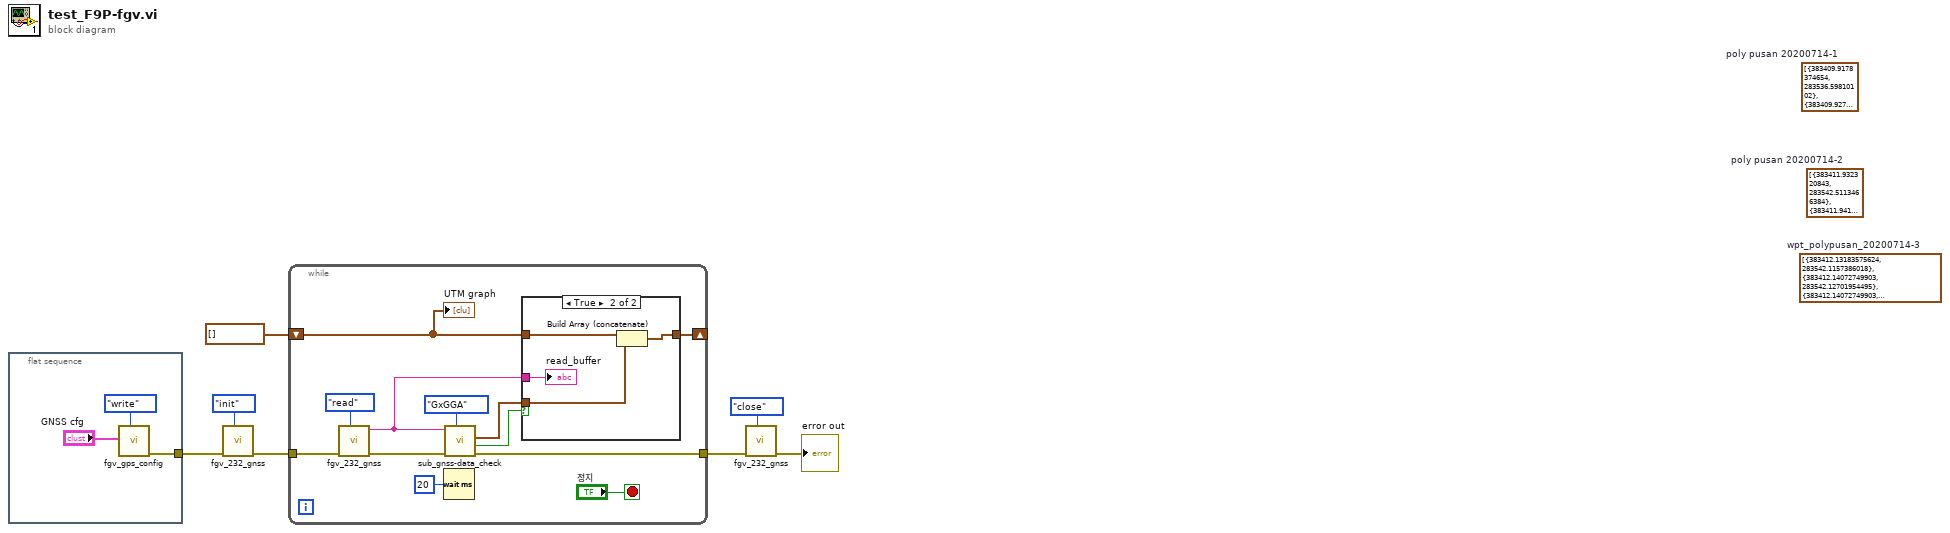
[diagram p0: block diagram]
diagram:
  (unwired) cluster{"X":dbl, "Y":dbl}[] [{"X"=383412.13183575624, "Y"=283542.1157386018}, {"X"=383412.14072749903, "Y"=283542.12701954495}, {"X"=383412.14072749903, "Y"=283542.12701954495}, {"X"=383412.14072749903, "Y"=283542.12701954495}, {"X"=383412.1496192395, "Y"=283542.1383004872}, {"X"=383412.1496192395, "Y"=283542.1383004872}, {"X"=383412.1496192395, "Y"=283542.1383004872}, {"X"=383412.1496192395, "Y"=283542.1383004872}, {"X"=383412.1496192395, "Y"=283542.1383004872}, {"X"=383412.1496192395, "Y"=283542.1383004872}, {"X"=383412.1589596947, "Y"=283542.1273881729}, {"X"=383412.1589596947, "Y"=283542.1273881729}, {"X"=383412.1589596947, "Y"=283542.1273881729}, {"X"=383412.1680757925, "Y"=283542.12757248693}, {"X"=383412.1683001499, "Y"=283542.11647585774}, {"X"=383412.1774162478, "Y"=283542.11666017177}, {"X"=383412.1774162478, "Y"=283542.11666017177}, {"X"=383412.1774162478, "Y"=283542.11666017177}, {"X"=383412.18675670295, "Y"=283542.10574785754}, {"X"=383412.18675670295, "Y"=283542.10574785754}, {"X"=383412.1958728009, "Y"=283542.1059321715}, {"X"=383412.1960971583, "Y"=283542.0948355424}, {"X"=383412.20521325845, "Y"=283542.09501985647}, {"X"=383412.20521325845, "Y"=283542.09501985647}, {"X"=383412.214329354, "Y"=283542.09520417044}, {"X"=383412.214329354, "Y"=283542.09520417044}, {"X"=383412.2234454518, "Y"=283542.0953884845}, {"X"=383412.2234454518, "Y"=283542.0953884845}, {"X"=383412.2234454518, "Y"=283542.0953884845}, {"X"=383412.214329354, "Y"=283542.09520417044}, {"X"=383412.214329354, "Y"=283542.09520417044}, {"X"=383412.214329354, "Y"=283542.09520417044}, {"X"=383412.2145537114, "Y"=283542.08410754264}, {"X"=383412.20543761586, "Y"=283542.08392322867}, {"X"=383412.2056619733, "Y"=283542.0728265995}, {"X"=383412.19654587307, "Y"=283542.07264228543}, {"X"=383412.19677023054, "Y"=283542.0615456572}, {"X"=383412.0980636525, "Y"=283541.9818418036}, {"X"=383411.97245749284, "Y"=283541.87939175277}, {"X"=383411.8288434909, "Y"=283541.76547644875}, {"X"=383411.64966251695, "Y"=283541.6064373785}, {"X"=383411.4077906293, "Y"=283541.390624976}, {"X"=383411.0658659977, "Y"=283541.16168851225}, {"X"=383410.6785852051, "Y"=283540.920733869}, {"X"=383410.30953659787, "Y"=283540.6801478684}, {"X"=383409.922704477, "Y"=283540.41700000333}, {"X"=383409.49985664326, "Y"=283540.1309216538}, {"X"=383409.04943613, "Y"=283539.85538702144}, {"X"=383408.5990155877, "Y"=283539.5798524129}, {"X"=383408.15771112393, "Y"=283539.30450213735}, {"X"=383407.7252983808, "Y"=283539.0404328218}, {"X"=383407.30200171185, "Y"=283538.7765478377}, {"X"=383406.8962641739, "Y"=283538.54632137535}, {"X"=383406.4998670677, "Y"=283538.3051826139}, {"X"=383406.10369428596, "Y"=283538.05294724106}, {"X"=383405.6895136327, "Y"=283537.7892466443}, {"X"=383405.28444905346, "Y"=283537.52573037276}, {"X"=383404.870044003, "Y"=283537.2731264438}, {"X"=383404.4554145847, "Y"=283537.0316191623}, {"X"=383404.04100949224, "Y"=283536.77901527355}, {"X"=383403.6266043726, "Y"=283536.52641140413}, {"X"=383403.18529961235, "Y"=283536.2510613829}, {"X"=383402.7346543793, "Y"=283535.9866237099}, {"X"=383402.29312522465, "Y"=283535.72237036366}, {"X"=383401.85182039154, "Y"=283535.44702041155}, {"X"=383401.43763949943, "Y"=283535.18332001864}, {"X"=383401.0603716887, "Y"=283534.89816360164}, {"X"=383400.74758961983, "Y"=283534.58100742893}, {"X"=383400.4815097676, "Y"=283534.2092896391}, {"X"=383400.280140006, "Y"=283533.79447545746}, {"X"=383400.14348033105, "Y"=283533.33656487794}, {"X"=383400.07197944535, "Y"=283532.81336464395}, {"X"=383400.0834208813, "Y"=283532.24743661174}, {"X"=383400.18602339644, "Y"=283531.68335159513}, {"X"=383400.41512973054, "Y"=283531.17732994177}, {"X"=383400.72426198516, "Y"=283530.7728366644}, {"X"=383401.0771800759, "Y"=283530.4580379334}, {"X"=383401.45587610855, "Y"=283530.2214685208}, {"X"=383401.88792276254, "Y"=283530.0525847101}, {"X"=383402.30928290833, "Y"=283529.9611930121}, {"X"=383402.7477535631, "Y"=283529.9256530838}, {"X"=383403.16642158024, "Y"=283529.9674209622}, {"X"=383403.52904686355, "Y"=283530.07466280117}, {"X"=383403.90878262615, "Y"=283530.2377564051}, {"X"=383404.31496931607, "Y"=283530.44578945445}, {"X"=383404.7382664643, "Y"=283530.7096742769}, {"X"=383405.1704553586, "Y"=283530.9848400567}, {"X"=383405.5937524603, "Y"=283531.2487249207}, {"X"=383405.99926602206, "Y"=283531.4900479345}, {"X"=383406.3954391052, "Y"=283531.7422832877}, {"X"=383406.81828743755, "Y"=283532.02836147026}, {"X"=383407.25002750533, "Y"=283532.3257206095}, {"X"=383407.6726514358, "Y"=283532.6228954618}, {"X"=383408.0954996884, "Y"=283532.9089737058}, {"X"=383408.5456962394, "Y"=283533.19560490194}, {"X"=383408.98655230104, "Y"=283533.4931484379}, {"X"=383409.40962482896, "Y"=283533.7681301187}, {"X"=383409.81446512, "Y"=283534.0427432001}, {"X"=383410.2101892815, "Y"=283534.3171719865}, {"X"=383410.6150295247, "Y"=283534.5917851032}, {"X"=383411.02898584673, "Y"=283534.86658255244}, {"X"=383411.4431665024, "Y"=283535.1302833934}, {"X"=383411.8575714911, "Y"=283535.3828876251}, {"X"=383412.28975995193, "Y"=283535.65805376216}, {"X"=383412.7401805953, "Y"=283535.9335885495}, {"X"=383413.1632529006, "Y"=283536.20857041556}, {"X"=383413.5772090795, "Y"=283536.48336798773}, {"X"=383414.00028133026, "Y"=283536.75834989623}, {"X"=383414.47737710393, "Y"=283537.0677276065}, {"X"=383414.95424848073, "Y"=283537.38820197195}, {"X"=383415.36775582953, "Y"=283537.6851928882}, {"X"=383415.72634217737, "Y"=283537.9921745477}, {"X"=383416.0202183364, "Y"=283538.3422525123}, {"X"=383416.2673921541, "Y"=283538.74689204094}, {"X"=383416.4496314275, "Y"=283539.2057244933}, {"X"=383416.54870396585, "Y"=283539.7183812282}, {"X"=383416.5472750222, "Y"=283540.24010709027}, {"X"=383416.48270647053, "Y"=283540.7272528411}, {"X"=383416.3369904831, "Y"=283541.1683532132}, {"X"=383416.1096783414, "Y"=283541.5856014671}, {"X"=383415.8103348771, "Y"=283541.95698867145}, {"X"=383415.43006836623, "Y"=283542.2712338854}, {"X"=383414.9873353622, "Y"=283542.51760912524}, {"X"=383414.50993287616, "Y"=283542.67447409057}, {"X"=383414.0436657404, "Y"=283542.73165373795}, {"X"=383413.5880852258, "Y"=283542.7113413258}, {"X"=383413.1160673846, "Y"=283542.60188727773}, {"X"=383412.6638522345, "Y"=283542.41512548324}, {"X"=383412.2316641198, "Y"=283542.1399593133}, {"X"=383412.1058336066, "Y"=283542.04860588827}, {"X"=383412.09671750874, "Y"=283542.04842157435}, {"X"=383412.1058336066, "Y"=283542.04860588827}, {"X"=383412.1149497068, "Y"=283542.04879020224}, {"X"=383412.12406580243, "Y"=283542.04897451616}, {"X"=383412.13295754296, "Y"=283542.0602554593}, {"X"=383412.13295754296, "Y"=283542.0602554593}, {"X"=383412.14207364316, "Y"=283542.06043977325}, {"X"=383412.1511897411, "Y"=283542.06062408723}, {"X"=383412.160305839, "Y"=283542.0608084012}]  # wpt_polypusan_20200714-3
  (unwired) cluster{"X":dbl, "Y":dbl}[] [{"X"=383411.932320843, "Y"=283542.5113466384}, {"X"=383411.94143694045, "Y"=283542.5115309522}, {"X"=383411.9503286807, "Y"=283542.5228118937}, {"X"=383411.95944477816, "Y"=283542.5229962075}, {"X"=383411.96856087557, "Y"=283542.5231805213}, {"X"=383411.9683365184, "Y"=283542.53427715093}, {"X"=383411.9774526181, "Y"=283542.5344614648}, {"X"=383411.9865687132, "Y"=283542.53464577853}, {"X"=383411.9956848153, "Y"=283542.5348300925}, {"X"=383411.8696299463, "Y"=283542.4545732997}, {"X"=383411.6993407283, "Y"=283542.3068151703}, {"X"=383411.54683498706, "Y"=283542.18161892693}, {"X"=383411.37654576113, "Y"=283542.0338608031}, {"X"=383411.1517842929, "Y"=283541.87390017736}, {"X"=383410.8998988804, "Y"=283541.7022899903}, {"X"=383410.62978125946, "Y"=283541.5303111862}, {"X"=383410.3509962426, "Y"=283541.33595482114}, {"X"=383410.072211214, "Y"=283541.1415984661}, {"X"=383409.7754183256, "Y"=283540.9357768668}, {"X"=383409.4697336811, "Y"=283540.71867434034}, {"X"=383409.146265533, "Y"=283540.47900994436}, {"X"=383408.83146475896, "Y"=283540.26172312885}, {"X"=383408.5526796635, "Y"=283540.0673668221}, {"X"=383408.28256195365, "Y"=283539.8953880912}, {"X"=383408.0122198793, "Y"=283539.7345059978}, {"X"=383407.7872339495, "Y"=283539.5856420879}, {"X"=383407.6249389544, "Y"=283539.4935514922}, {"X"=383407.4177365061, "Y"=283539.36724946724}, {"X"=383407.18341010157, "Y"=283539.2292978924}, {"X"=383406.9399675942, "Y"=283539.0911620164}, {"X"=383406.6513932718, "Y"=283538.92991135013}, {"X"=383406.33591933665, "Y"=283538.74591451185}, {"X"=383405.98465403315, "Y"=283538.5278905661}, {"X"=383405.6333887108, "Y"=283538.3098666383}, {"X"=383405.2641155198, "Y"=283538.080377482}, {"X"=383404.8590509454, "Y"=283537.8168612309}, {"X"=383404.4450945958, "Y"=283537.54206406383}, {"X"=383404.04025432153, "Y"=283537.2674512232}, {"X"=383403.6443057818, "Y"=283537.00411933445}, {"X"=383403.2485815608, "Y"=283536.7296908353}, {"X"=383402.85263297544, "Y"=283536.4663589834}, {"X"=383402.4389008485, "Y"=283536.18046528485}, {"X"=383402.025168696, "Y"=283535.89457160764}, {"X"=383401.6474522479, "Y"=283535.6316084193}, {"X"=383401.2877436384, "Y"=283535.38011048}, {"X"=383400.94694025436, "Y"=283535.0956912774}, {"X"=383400.62571511255, "Y"=283534.74506092304}, {"X"=383400.3509678404, "Y"=283534.35096557817}, {"X"=383400.140930653, "Y"=283533.9137738416}, {"X"=383399.99582789536, "Y"=283533.42238907877}, {"X"=383399.9518996638, "Y"=283532.8886451223}, {"X"=383399.9995811818, "Y"=283532.33455092355}, {"X"=383400.1475398879, "Y"=283531.782484042}, {"X"=383400.4042188871, "Y"=283531.26591866364}, {"X"=383400.7318076984, "Y"=283530.8506973626}, {"X"=383401.120965875, "Y"=283530.54773247044}, {"X"=383401.56325033365, "Y"=283530.32354980666}, {"X"=383402.03998015146, "Y"=283530.1999740305}, {"X"=383402.5151395754, "Y"=283530.15407467587}, {"X"=383402.9796124794, "Y"=283530.1856674368}, {"X"=383403.4247314314, "Y"=283530.2723747546}, {"X"=383403.85004773084, "Y"=283530.4363898795}, {"X"=383404.2922501598, "Y"=283530.6673534074}, {"X"=383404.74311997613, "Y"=283530.92069452035}, {"X"=383405.16664144257, "Y"=283531.17348273523}, {"X"=383405.61751120875, "Y"=283531.42682389263}, {"X"=383406.08594012377, "Y"=283531.7138235732}, {"X"=383406.5452528999, "Y"=283532.00063897157}, {"X"=383407.04013267846, "Y"=283532.33257814153}, {"X"=383407.5619120408, "Y"=283532.6872635217}, {"X"=383408.092583116, "Y"=283533.0532298735}, {"X"=383408.5968032415, "Y"=283533.37425681524}, {"X"=383409.08279111754, "Y"=283533.69491516484}, {"X"=383409.5692276718, "Y"=283533.9933802838}, {"X"=383410.10057165544, "Y"=283534.3260568743}, {"X"=383410.6854904599, "Y"=283534.7153225135}, {"X"=383411.26106875925, "Y"=283535.11550050834}, {"X"=383411.8279796103, "Y"=283535.493300969}, {"X"=383412.34998296807, "Y"=283535.83689001354}, {"X"=383412.82707883895, "Y"=283536.14626763324}, {"X"=383413.3495308398, "Y"=283536.4676634827}, {"X"=383413.89021501347, "Y"=283536.7894279925}, {"X"=383414.3762025273, "Y"=283537.11008664395}, {"X"=383414.844182165, "Y"=283537.4192800597}, {"X"=383415.32082914957, "Y"=283537.7508510744}, {"X"=383415.7781220907, "Y"=283538.1375366228}, {"X"=383416.1426834359, "Y"=283538.6000554199}, {"X"=383416.40562146157, "Y"=283539.12712650327}, {"X"=383416.53981222806, "Y"=283539.7071002825}, {"X"=383416.57305278804, "Y"=283540.31833644706}, {"X"=383416.451319649, "Y"=283540.92643920117}, {"X"=383416.2213151491, "Y"=283541.47684699734}, {"X"=383415.8748206522, "Y"=283541.92498900933}, {"X"=383415.43006836623, "Y"=283542.2712338854}, {"X"=383414.93241441366, "Y"=283542.5275998535}, {"X"=383414.4092070801, "Y"=283542.694639868}, {"X"=383413.8978081814, "Y"=283542.7287046846}, {"X"=383413.33350757346, "Y"=283542.6728906116}, {"X"=383412.79879883706, "Y"=283542.50666323025}, {"X"=383412.3112410692, "Y"=283542.2636810541}, {"X"=383412.1309383268, "Y"=283542.1601251152}, {"X"=383412.1222709437, "Y"=283542.13774754526}, {"X"=383412.1222709437, "Y"=283542.13774754526}, {"X"=383412.1316113989, "Y"=283542.12683523097}, {"X"=383412.1316113989, "Y"=283542.12683523097}, {"X"=383412.1316113989, "Y"=283542.12683523097}, {"X"=383412.1316113989, "Y"=283542.12683523097}, {"X"=383412.1316113989, "Y"=283542.12683523097}, {"X"=383412.14072749903, "Y"=283542.12701954495}, {"X"=383412.14984359685, "Y"=283542.1272038589}]  # poly pusan 20200714-2
  (unwired) cluster{"X":dbl, "Y":dbl}[] [{"X"=383409.9178374654, "Y"=283536.59810102}, {"X"=383409.927177923, "Y"=283536.58718870144}, {"X"=383409.93651838053, "Y"=283536.57627638616}, {"X"=383409.9549749438, "Y"=283536.5655483811}, {"X"=383409.96431539906, "Y"=283536.55463606486}, {"X"=383409.973655859, "Y"=283536.5437237469}, {"X"=383409.98277195997, "Y"=283536.54390805843}, {"X"=383409.9469806094, "Y"=283536.50988092675}, {"X"=383409.93831321446, "Y"=283536.4875033598}, {"X"=383409.9385375687, "Y"=283536.4764067302}, {"X"=383409.9385375687, "Y"=283536.4764067302}, {"X"=383409.93876192294, "Y"=283536.4653101011}, {"X"=383409.8578387605, "Y"=283536.40816815686}, {"X"=383409.7769156017, "Y"=283536.35102621204}, {"X"=383409.7589077463, "Y"=283536.3395609602}, {"X"=383409.73200814123, "Y"=283536.3168147713}, {"X"=383409.5792779161, "Y"=283536.20271519583}, {"X"=383409.27336874546, "Y"=283535.99670931126}, {"X"=383408.841180219, "Y"=283535.72154332086}, {"X"=383408.3816433538, "Y"=283535.4458244228}, {"X"=383408.05727756815, "Y"=283535.25054659066}, {"X"=383407.9223308085, "Y"=283535.15900892194}, {"X"=383407.94056302006, "Y"=283535.15937754087}, {"X"=383408.09396634065, "Y"=283535.2401872}, {"X"=383408.3194010837, "Y"=283535.36685785564}, {"X"=383408.61776466237, "Y"=283535.4950029968}, {"X"=383409.05421591504, "Y"=283535.55933303706}, {"X"=383409.60140653874, "Y"=283535.55929506075}, {"X"=383410.21285860625, "Y"=283535.5383540437}, {"X"=383410.69646085746, "Y"=283535.52592932346}, {"X"=383410.96971964114, "Y"=283535.5425553223}, {"X"=383411.1155773138, "Y"=283535.5455043238}, {"X"=383411.3519229675, "Y"=283535.5835863414}, {"X"=383411.5695876939, "Y"=283535.64349299634}, {"X"=383411.6963157314, "Y"=283535.69045989437}, {"X"=383411.94954744837, "Y"=283535.7954903261}, {"X"=383412.0940589766, "Y"=283535.86501911347}, {"X"=383412.17520648835, "Y"=283535.9110644512}, {"X"=383412.2472378928, "Y"=283535.95692547486}, {"X"=383412.2743618502, "Y"=283535.9685750442}, {"X"=383412.2743618502, "Y"=283535.9685750442}, {"X"=383412.2741374931, "Y"=283535.9796716734}, {"X"=383412.2741374931, "Y"=283535.9796716734}, {"X"=383412.2741374931, "Y"=283535.9796716734}, {"X"=383412.2741374931, "Y"=283535.9796716734}, {"X"=383412.2741374931, "Y"=283535.9796716734}, {"X"=383412.2741374931, "Y"=283535.9796716734}, {"X"=383412.2741374931, "Y"=283535.9796716734}, {"X"=383412.2741374931, "Y"=283535.9796716734}, {"X"=383412.2743618502, "Y"=283535.9685750442}, {"X"=383412.26524574624, "Y"=283535.9683907304}, {"X"=383412.2650213891, "Y"=283535.9794873595}, {"X"=383412.2650213891, "Y"=283535.9794873595}, {"X"=383412.2559052828, "Y"=283535.97930304566}, {"X"=383412.291920987, "Y"=283536.0022335576}, {"X"=383412.53581222554, "Y"=283536.11817631975}, {"X"=383412.77970346273, "Y"=283536.2341190897}, {"X"=383412.987578986, "Y"=283536.3271313491}, {"X"=383413.19545451214, "Y"=283536.42014361545}, {"X"=383413.367089974, "Y"=283536.5013219984}, {"X"=383413.49336927186, "Y"=283536.5704821794}, {"X"=383413.5293849731, "Y"=283536.59341269743}, {"X"=383413.5385010765, "Y"=283536.5935970126}, {"X"=383413.5567332834, "Y"=283536.5939656429}, {"X"=383413.56584938685, "Y"=283536.59414995805}, {"X"=383413.5749654926, "Y"=283536.59433427325}, {"X"=383413.71013653226, "Y"=283536.6747754009}, {"X"=383414.22324801044, "Y"=283537.0070836166}, {"X"=383414.9242078476, "Y"=283537.5208085642}, {"X"=383415.63002084335, "Y"=283538.2455538307}, {"X"=383416.1836939611, "Y"=283539.2780556692}, {"X"=383416.2779721501, "Y"=283540.4788876928}, {"X"=383415.9344532047, "Y"=283541.68196908606}, {"X"=383415.1402897733, "Y"=283542.62061217}, {"X"=383414.0938751328, "Y"=283542.95469220664}, {"X"=383413.47308307973, "Y"=283542.9865452564}, {"X"=383413.3452333581, "Y"=283542.9950614707}, {"X"=383413.3267768075, "Y"=283543.0057894686}, {"X"=383413.3174363517, "Y"=283543.01670178166}, {"X"=383413.38102467154, "Y"=283543.0290886174}, {"X"=383413.9084121501, "Y"=283543.1063586886}, {"X"=383414.70860945265, "Y"=283543.2224481709}, {"X"=383414.95384662825, "Y"=283543.2718112374}, {"X"=383414.95362226735, "Y"=283543.2829078666}, {"X"=383414.9533979065, "Y"=283543.2940044949}, {"X"=383414.9531735456, "Y"=283543.3051011227}, {"X"=383414.9169335171, "Y"=283543.29326722753}, {"X"=383414.6076593038, "Y"=283543.25371057465}, {"X"=383413.9711030325, "Y"=283543.1631320421}, {"X"=383413.3634655521, "Y"=283542.9954301012}, {"X"=383412.93972051237, "Y"=283542.7537380956}, {"X"=383412.5989177596, "Y"=283542.4693184259}, {"X"=383412.09537136485, "Y"=283542.11500134604}, {"X"=383411.53690398356, "Y"=283541.77067504416}, {"X"=383411.0869323256, "Y"=283541.47294704843}, {"X"=383410.7814720845, "Y"=283541.2447478443}, {"X"=383410.583610174, "Y"=283541.1075334294}, {"X"=383410.466222666, "Y"=283541.04965422716}, {"X"=383410.4297582683, "Y"=283541.04891697824}, {"X"=383410.41130171315, "Y"=283541.059644982}, {"X"=383410.8434899318, "Y"=283541.33481106185}, {"X"=383411.3746090679, "Y"=283541.67858437833}, {"X"=383411.8963877096, "Y"=283542.03327004256}, {"X"=383412.49042201624, "Y"=283542.42272013833}, {"X"=383413.04044630117, "Y"=283542.7335723024}, {"X"=383413.4459591501, "Y"=283542.9748956804}, {"X"=383413.81545630284, "Y"=283543.1932885606}, {"X"=383414.26654959243, "Y"=283543.4355335569}, {"X"=383414.59158803057, "Y"=283543.59752174537}, {"X"=383414.6727354587, "Y"=283543.6435671087}, {"X"=383414.6725110981, "Y"=283543.65466373705}, {"X"=383414.663395004, "Y"=283543.6544794205}, {"X"=383414.5277753554, "Y"=283543.59623153013}, {"X"=383414.39215570525, "Y"=283543.53798364184}, {"X"=383414.1751642665, "Y"=283543.4447870245}, {"X"=383413.7863131391, "Y"=283543.2815086416}, {"X"=383413.42548336374, "Y"=283543.085493336}, {"X"=383413.1546927557, "Y"=283542.94680433837}, {"X"=383412.9650495782, "Y"=283542.854160697}, {"X"=383412.7938629567, "Y"=283542.75078906}, {"X"=383412.56865281187, "Y"=283542.6130216534}, {"X"=383412.41547401866, "Y"=283542.52111528144}, {"X"=383412.37056660216, "Y"=283542.48690382455}, {"X"=383412.36167486466, "Y"=283542.47562288266}, {"X"=383412.28120048554, "Y"=283542.39628765377}, {"X"=383412.2182852302, "Y"=283542.3506109417}, {"X"=383412.2091691326, "Y"=283542.3504266277}, {"X"=383412.2093934901, "Y"=283542.33932999894}, {"X"=383412.2093934901, "Y"=283542.33932999894}, {"X"=383412.2093934901, "Y"=283542.33932999894}, {"X"=383412.2093934901, "Y"=283542.33932999894}, {"X"=383412.2463065955, "Y"=283542.3178739988}, {"X"=383412.2554226954, "Y"=283542.31805831287}, {"X"=383412.2645387931, "Y"=283542.31824262696}, {"X"=383412.2738792506, "Y"=283542.3073303115}, {"X"=383412.1665052908, "Y"=283542.2052488859}, {"X"=383411.77922457363, "Y"=283541.9642941928}, {"X"=383411.38305209693, "Y"=283541.71205857664}, {"X"=383411.10381838854, "Y"=283541.5398954449}, {"X"=383410.8697164487, "Y"=283541.3908471426}, {"X"=383410.6447306024, "Y"=283541.2419831568}, {"X"=383410.41062864766, "Y"=283541.0929348684}, {"X"=383410.14940274344, "Y"=283540.9322370196}, {"X"=383409.9155251322, "Y"=283540.77209211467}, {"X"=383409.6903149036, "Y"=283540.6343247839}, {"X"=383409.43842942733, "Y"=283540.4627146399}, {"X"=383409.24056747806, "Y"=283540.3255002548}, {"X"=383409.17765219585, "Y"=283540.27982356516}, {"X"=383409.2585753234, "Y"=283540.3369655045}, {"X"=383409.5375847504, "Y"=283540.52022520616}, {"X"=383409.8617259532, "Y"=283540.7265997316}, {"X"=383410.20365063194, "Y"=283540.95553614816}, {"X"=383410.608939274, "Y"=283541.20795602264}, {"X"=383410.995546983, "Y"=283541.4822005473}, {"X"=383411.3283555053, "Y"=283541.7109526976}, {"X"=383411.68873666425, "Y"=283541.9291611722}, {"X"=383411.95862989506, "Y"=283542.1122366382}, {"X"=383412.12070044235, "Y"=283542.2154239456}, {"X"=383412.1567161209, "Y"=283542.2383544585}, {"X"=383412.1658322186, "Y"=283542.23853877245}, {"X"=383412.1658322186, "Y"=283542.23853877245}, {"X"=383412.1749483163, "Y"=283542.2387230865}, {"X"=383412.1749483163, "Y"=283542.2387230865}, {"X"=383412.2025209692, "Y"=283542.2281793989}, {"X"=383412.2025209692, "Y"=283542.2281793989}, {"X"=383412.2025209692, "Y"=283542.2281793989}, {"X"=383412.21163706464, "Y"=283542.22836371296}, {"X"=383412.21163706464, "Y"=283542.22836371296}, {"X"=383412.22052880493, "Y"=283542.2396446566}, {"X"=383412.22052880493, "Y"=283542.2396446566}, {"X"=383412.18496184365, "Y"=283542.1945208857}, {"X"=383412.09537136485, "Y"=283542.11500134604}, {"X"=383411.9788813051, "Y"=283542.0127356099}, {"X"=383411.8530507877, "Y"=283541.9213821895}, {"X"=383411.67274803354, "Y"=283541.8178262597}, {"X"=383411.46532133967, "Y"=283541.7026207666}, {"X"=383411.29413467535, "Y"=283541.59924916073}, {"X"=383411.1767471755, "Y"=283541.54136994836}, {"X"=383411.07759187114, "Y"=283541.48385936284}, {"X"=383410.9510882701, "Y"=283541.42579584295}, {"X"=383410.80702553515, "Y"=283541.33407381136}, {"X"=383410.6173823041, "Y"=283541.24143021955}, {"X"=383410.48198695586, "Y"=283541.1720857659}, {"X"=383410.4457469139, "Y"=283541.16025188734}, {"X"=383410.43663081515, "Y"=283541.1600675751}, {"X"=383410.3557076998, "Y"=283541.1029256232}, {"X"=383410.1934127563, "Y"=283541.0108349785}, {"X"=383410.0039938697, "Y"=283540.90709477285}, {"X"=383409.7696675421, "Y"=283540.769143129}, {"X"=383409.53511685575, "Y"=283540.6422881183}, {"X"=383409.3730462501, "Y"=283540.53910085984}, {"X"=383409.2380995876, "Y"=283540.44756316737}, {"X"=383409.04912938597, "Y"=283540.3216297263}, {"X"=383408.81480303186, "Y"=283540.1836781074}, {"X"=383408.55402578035, "Y"=283540.00078705046}, {"X"=383408.26590022095, "Y"=283539.817343072}, {"X"=383407.9686585453, "Y"=283539.63371479337}, {"X"=383407.67141686263, "Y"=283539.450086526}, {"X"=383407.3743995172, "Y"=283539.2553616379}, {"X"=383407.05025820807, "Y"=283539.0489872076}, {"X"=383406.71700078365, "Y"=283538.8424284801}, {"X"=383406.3926350932, "Y"=283538.64715070394}, {"X"=383406.04159413883, "Y"=283538.41803012847}, {"X"=383405.7174527709, "Y"=283538.2116557487}, {"X"=383405.4113192408, "Y"=283538.01674662315}, {"X"=383405.0869534989, "Y"=283537.8214688956}, {"X"=383404.7810442931, "Y"=283537.615463163}, {"X"=383404.4840268283, "Y"=283537.4207383768}, {"X"=383404.21413331095, "Y"=283537.2376631467}, {"X"=383403.9440154383, "Y"=283537.06568455126}, {"X"=383403.65588969685, "Y"=283536.8822407282}, {"X"=383403.36753959535, "Y"=283536.70989354217}, {"X"=383403.0525142093, "Y"=283536.5037035683}, {"X"=383402.692581331, "Y"=283536.26330219803}, {"X"=383402.3237566754, "Y"=283536.0116199123}, {"X"=383401.990947726, "Y"=283535.7828681109}, {"X"=383401.75729418325, "Y"=283535.61162680085}, {"X"=383401.6312391361, "Y"=283535.5313701584}, {"X"=383401.4962923195, "Y"=283535.4398325877}, {"X"=383401.2984301499, "Y"=283535.30261838617}, {"X"=383401.0827844499, "Y"=283535.1428423272}, {"X"=383400.8944870562, "Y"=283534.98361918115}, {"X"=383400.70641399856, "Y"=283534.8132994113}, {"X"=383400.5010060944, "Y"=283534.5982245295}, {"X"=383400.3060603416, "Y"=283534.3167541855}, {"X"=383400.13958460063, "Y"=283533.9803536106}, {"X"=383400.00157887576, "Y"=283533.5890228039}, {"X"=383399.91049971955, "Y"=283533.1320337348}, {"X"=383399.89302243193, "Y"=283532.64322919585}, {"X"=383399.93890921294, "Y"=283532.17790802126}, {"X"=383400.04703835654, "Y"=283531.79155335313}, {"X"=383400.18049675727, "Y"=283531.50562124373}, {"X"=383400.30304432334, "Y"=283531.3082778588}, {"X"=383400.38800574763, "Y"=283531.1656804091}, {"X"=383400.50053984235, "Y"=283531.0125392357}, {"X"=383400.68712452496, "Y"=283530.8053893417}, {"X"=383400.8917170911, "Y"=283530.60970468115}, {"X"=383401.1596737439, "Y"=283530.43750339915}, {"X"=383401.4545300481, "Y"=283530.2880482896}, {"X"=383401.78517776896, "Y"=283530.17262028495}, {"X"=383402.16984912794, "Y"=283530.09158799663}, {"X"=383402.58052275726, "Y"=283530.07768840576}, {"X"=383402.9811828962, "Y"=283530.1079910402}, {"X"=383403.37115650147, "Y"=283530.2157857858}, {"X"=383403.8138076402, "Y"=283530.42455603235}, {"X"=383404.3193741375, "Y"=283530.6790029523}, {"X"=383404.7793600638, "Y"=283530.93252837134}, {"X"=383405.14863357117, "Y"=283531.1620174932}, {"X"=383405.4187516078, "Y"=283531.3339961164}, {"X"=383405.5988302973, "Y"=283531.4486485354}, {"X"=383405.77868462657, "Y"=283531.5743975866}, {"X"=383405.95876330684, "Y"=283531.6890500145}, {"X"=383406.19264122855, "Y"=283531.8491948027}, {"X"=383406.51633412845, "Y"=283532.0777624464}, {"X"=383406.8495918177, "Y"=283532.2843211534}, {"X"=383407.1286015494, "Y"=283532.4675807652}, {"X"=383407.4076112677, "Y"=283532.650840386}, {"X"=383407.70485319116, "Y"=283532.83446863596}, {"X"=383408.00187074905, "Y"=283533.0291935228}, {"X"=383408.3353527256, "Y"=283533.2246556581}, {"X"=383408.66838598094, "Y"=283533.44231106626}, {"X"=383408.97474396054, "Y"=283533.6261236677}, {"X"=383409.27176146646, "Y"=283533.8208486002}, {"X"=383409.61368643295, "Y"=283534.04978498194}, {"X"=383410.0009675565, "Y"=283534.2907395623}, {"X"=383410.39736476535, "Y"=283534.5318784738}, {"X"=383410.76641363365, "Y"=283534.7724644647}, {"X"=383411.117454633, "Y"=283535.0015852203}, {"X"=383411.4778360758, "Y"=283535.2197936726}, {"X"=383411.8831249549, "Y"=283535.4722135931}, {"X"=383412.2695085299, "Y"=283535.75755479146}, {"X"=383412.6385573031, "Y"=283535.9981408621}, {"X"=383412.9624742541, "Y"=283536.21561212145}, {"X"=383413.2866155505, "Y"=283536.4219867639}, {"X"=383413.62876467826, "Y"=283536.6398266781}, {"X"=383413.9800298931, "Y"=283536.85785092146}, {"X"=383414.3404111968, "Y"=283537.0760594928}, {"X"=383414.6736685308, "Y"=283537.28261850367}, {"X"=383414.979801905, "Y"=283537.47752794967}, {"X"=383415.28571090545, "Y"=283537.6835340353}, {"X"=383415.5911711697, "Y"=283537.91173338844}, {"X"=383415.88616914465, "Y"=283538.20632820437}, {"X"=383416.1620374513, "Y"=283538.5449409112}, {"X"=383416.38231168006, "Y"=283538.92683423456}, {"X"=383416.54744055454, "Y"=283539.3298149099}, {"X"=383416.64808362443, "Y"=283539.764795244}, {"X"=383416.66623305104, "Y"=283540.22030997305}, {"X"=383416.6021132184, "Y"=283540.6852624638}, {"X"=383416.4381650218, "Y"=283541.1259941986}, {"X"=383416.22930943617, "Y"=283541.53251445986}, {"X"=383415.9393064278, "Y"=283541.89298934815}, {"X"=383415.58638820087, "Y"=283542.2077875092}, {"X"=383415.21680833364, "Y"=283542.4445406474}, {"X"=383414.83945855283, "Y"=283542.6145297139}, {"X"=383414.4547875691, "Y"=283542.6955614495}, {"X"=383414.0258822629, "Y"=283542.70909185003}, {"X"=383413.5434021757, "Y"=283542.6660332347}, {"X"=383413.0713843318, "Y"=283542.55657918955}, {"X"=383412.6456200371, "Y"=283542.41475685424}, {"X"=383412.2850145638, "Y"=283542.2076449687}, {"X"=383412.1767431755, "Y"=283542.1499500583}, {"X"=383412.1767431755, "Y"=283542.1499500583}, {"X"=383412.1767431755, "Y"=283542.1499500583}, {"X"=383412.17651881813, "Y"=283542.1610466851}, {"X"=383412.17651881813, "Y"=283542.1610466851}]  # poly pusan 20200714-1
  n1 = flat-sequence {
    tunnel: [w9] -> w2
    frame #0 {
      n2 = call "fgv_gps_config.vi"("cmd"=enum16{"read", "write"}."write", "GNSS cfg"="GNSS cfg") -> ("error out"=w9:errorcluster)  [unwired: 8 in, 1 out]
    }
  }
  n3 = call "fgv_232_gnss.vi"("cmd"=enum16{"init", "read", "write", "close"}."init", "error in"=w2) -> ("error out"=w6:errorcluster)  [unwired: 7 in, 2 out]
  n4 = while {
    shift-right: [w20] -> _
    shift-left: cluster{"Y(E)":dbl, "X(N)":dbl}[] [] -> [w17]
    tunnel: w6 -> [w18]
    tunnel: [w11] -> w4
    stop <- "정지" stop-if-true
    n5 = call "fgv_232_gnss.vi"("cmd"=enum16{"init", "read", "write", "close"}."read", "error in"=w18) -> ("error out"=w12:errorcluster, "read_buffer"=w14:string)  [unwired: 7 in, 1 out]
    n6 = Wait (ms)(milliseconds to wait=u32 20 ("대기 시간 (ms)")) -> ()  [unwired: 1 out]
    n7 = call "sub_gnss-data_check.vi"("sel"=T2."GxGGA", "error in"=w12, "gnss str"=w14) -> ("error out"=w11:errorcluster, "val"=w16:bool, "TM"=w13:cluster{dbl, dbl})  [unwired: 5 in, 1 out]
    n8 = case shown="True" w16 {
      tunnel: [w23 w27] -> w20
      tunnel: w17 -> [w23 w26]
      tunnel: w14 -> [_ w25]
      tunnel: w13 -> [_ w24]
      frame False {
      }
      frame True {
        n9 = Build Array (concatenate)(w26, w24) -> (w27:cluster{"Y(E)":dbl, "X(N)":dbl}[])
        "read_buffer" <- w25
      }
    }
    "UTM graph" <- w17
  }
  n10 = call "fgv_232_gnss.vi"("cmd"=enum16{"init", "read", "write", "close"}."close", "error in"=w4) -> ("error out"=→"error out":errorcluster)  [unwired: 7 in, 2 out]
